vi "Sensitive Joystick.vi"(1 "Sensitivity":dbl, 2 "Joystick In":dbl) -> (0 "Joystick Out":dbl)   [LabVIEW 2015]
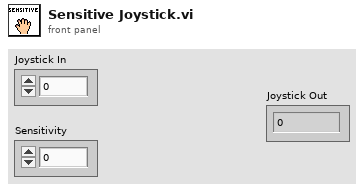
[diagram p1: front panel]
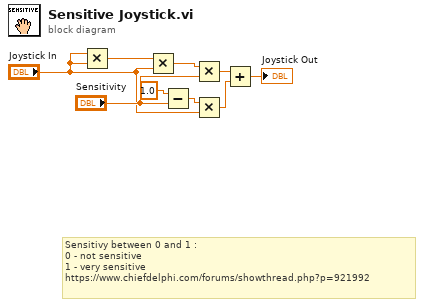
[diagram p0: block diagram]
diagram:
  # "Sensitivy between 0 and 1 :\n0 - not sensitive\n1 - very sensitive\nhttps://www.chiefdelphi.com/forums/showthread.php?p=921992"
  n1 = Multiply(x="Joystick In", y="Joystick In") -> (x*y=w9:dbl)
  n2 = Multiply(x=w9, y="Joystick In") -> (x*y=w1:dbl)
  n3 = Subtract(x=1.0, y="Sensitivity") -> (x-y=w7:dbl)
  n4 = Multiply(x=w1, y="Sensitivity") -> (x*y=w5:dbl)
  n5 = Multiply(x=w7, y="Joystick In") -> (x*y=w4:dbl)
  n6 = Add(x=w5, y=w4) -> (x+y=→"Joystick Out":dbl)
